vi "PUT (Buffer).vi"(6 "timeout":i32=10000, 7 "output file":path, 8 "error in":errorcluster, 9 "buffer":string, 10 "url":string, 11 "Session In":refnum<class "Session.lvclass">) -> (0 "error out":errorcluster, 1 "body":string, 2 "headers":string, 3 "Session Out":refnum<class "Session.lvclass">, 4 "status code":u32)   [LabVIEW 2020, in "Library Commun.lvlib" / "Library Http.lvlib" / "Session.lvclass"]
uses:
  Session.lvclass
  Session.lvclass/Session.ctl
  lvwebclient_32.dll
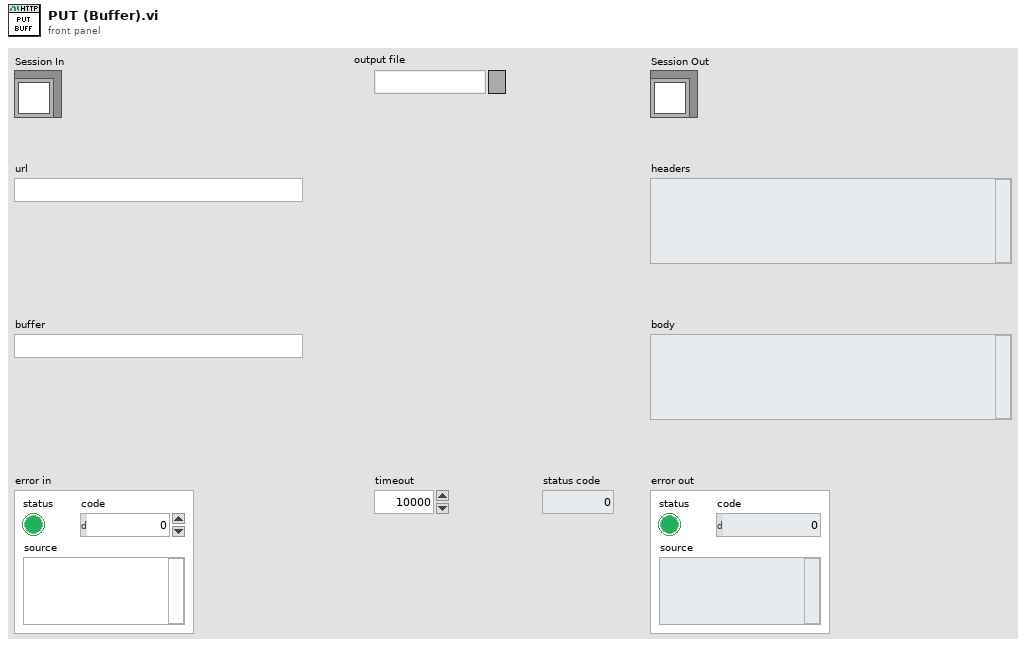
[diagram p1: front panel]
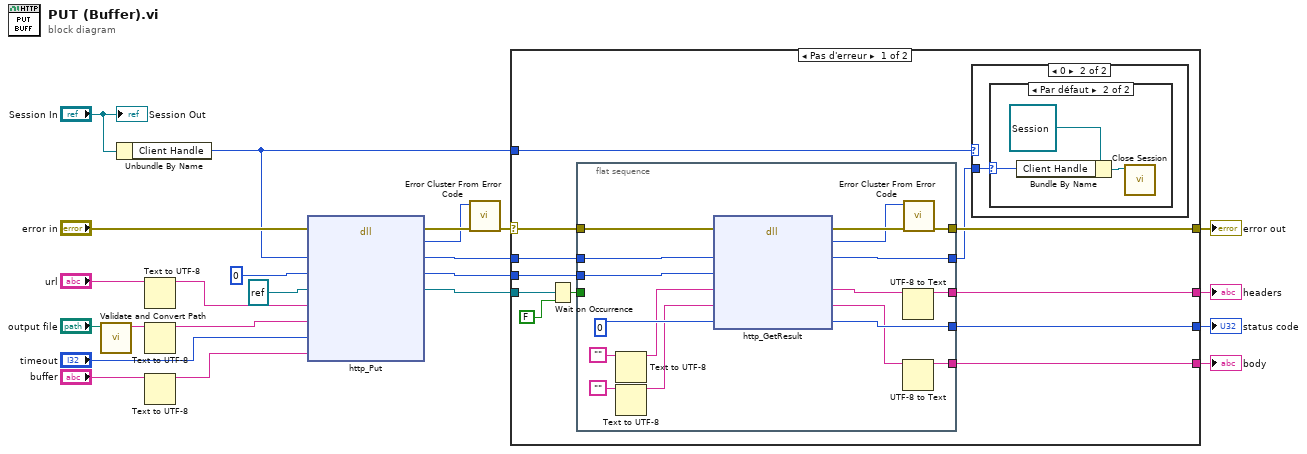
[diagram p0: block diagram]
diagram:
  n1 = call "Validate and Convert Path.vi"("path"="output file") -> ("validated path as string"=w15:string)  [unwired: 10 in]
  n2 = Unbundle By Name("Session In") -> ("Client Handle"=w10:u32)
  n3 = Text to UTF-8(11:"url") -> (3:w4:string)  [unwired: 2 in, 1 out]
  n4 = Text to UTF-8(11:w15) -> (3:w3:string)  [unwired: 2 in, 1 out]
  n5 = Text to UTF-8(11:"buffer") -> (3:w1:string)  [unwired: 2 in, 1 out]
  n6 = dll-call lib="C:/Users/ngarcin/OneDrive - Altyor/Standard TB/Class/Http Altyor/lvwebclient_*.*" fn="http_Put"(error in="error in", "handle"=w10, "request"=u32 0, "completeOccurrence"=refnum<k4> refnum ("occurrence"), "url"=w4, "outPath"=w3, "timeout"="timeout", "putData"=w1) -> (error out=w12:errorcluster, "return"=w11:i32, "handle"=w8:u32, "request"=w7:u32, "completeOccurrence"=w5:refnum<k4>)  [unwired: 6 in, 1 out]
  n7 = call <vilib>:"Error Cluster From Error Code.vi"("error in (no error)"=w12, "error code (0)"=w11) -> ("error out"=w23:errorcluster)  [unwired: 7 in]
  n8 = case shown="Pas d'erreur" w23 {
    selector: w23 -> [w33 w57]
    tunnel: w5 -> [w35 _]
    tunnel: w8 -> [w32 _]
    tunnel: w7 -> [w31 _]
    tunnel: [w30 _] -> w20
    tunnel: [w29 _] -> w19
    tunnel: [w28 _] -> w18
    tunnel: [w27 w57] -> w17
    tunnel: w10 -> [w26 _]
    frame No Error {
      n9 = Wait on Occurrence(1:FALSE, 2:w35) -> (0:w34:bool)  [unwired: 1 in]
      n10 = flat-sequence {
        tunnel: w34 -> [_]
        tunnel: w33 -> [w56]
        tunnel: w32 -> [w55]
        tunnel: w31 -> [w54]
        tunnel: [w52] -> w30
        tunnel: [w47] -> w29
        tunnel: [w46] -> w28
        tunnel: [w45] -> w27
        tunnel: [w44] -> w25
        frame #0 {
          n11 = Text to UTF-8(11:"") -> (3:w41:string)  [unwired: 2 in, 1 out]
          n12 = Text to UTF-8(11:"") -> (3:w40:string)  [unwired: 2 in, 1 out]
          n13 = dll-call lib="C:/Users/ngarcin/OneDrive - Altyor/Standard TB/Class/Http Altyor/lvwebclient_*.*" fn="http_GetResult"(error in=w56, "handle"=w55, "request"=w54, "returnHeader"=w41, "returnBody"=w40, "httpStatus"=u32 0) -> (error out=w51:errorcluster, "return"=w50:i32, "handle"=w44:u32, "returnHeader"=w49:string, "returnBody"=w48:string, "httpStatus"=w52:u32)  [unwired: 3 in, 1 out]
          n14 = UTF-8 to Text(11:w49) -> (3:w47:string)  [unwired: 2 in, 1 out]
          n15 = UTF-8 to Text(11:w48) -> (3:w46:string)  [unwired: 2 in, 1 out]
          n16 = call <vilib>:"Error Cluster From Error Code.vi"("error in (no error)"=w51, "error code (0)"=w50) -> ("error out"=w45:errorcluster)  [unwired: 7 in]
        }
      }
      n17 = case shown="0" w26 {
        tunnel: w25 -> [_ w36]
        frame Default {
        }
        frame 0 {
          n18 = case shown="Par défaut" w36 {
            selector: w36 -> [_ w39]
            frame 0 {
            }
            frame Default {
              n19 = Bundle By Name(cluster=refnum<class "Session.lvclass"> refnum ("Session Out"), "Client Handle"=w39) -> (w38:refnum<class "Session.lvclass">)
              n20 = call "Close Session.vi"("Session In"=w38) -> ()  [unwired: 10 in, 1 out]
            }
          }
        }
      }
    }
    frame Error {
    }
  }
  "error out" <- w17
  "headers" <- w19
  "body" <- w18
  "status code" <- w20
  "Session Out" <- "Session In"
